vi "format_streaming_channels.set.vi"(8 "error in":errorcluster, 9 "paths":string[](array[string]), 10 "names":string[](array[string]), 11 "Nominal IO Client in":T1 format="%.0x") -> (0 "error out":errorcluster, 1 "saved paths":string[](array[string]), 2 "saved names":string[](array[string]), 3 "Nominal IO Client out":T1 format="%.0x")   [LabVIEW 2024, in "Nominal Client Scripting.lvlib"]
uses:
  Nominal Client Scripting.lvlib
  <vilib>/NI VeriStand/Custom Device API/Custom Device Item Ref.ctl
  <vilib>/NI VeriStand/Custom Device API/Custom Device API.lvlib
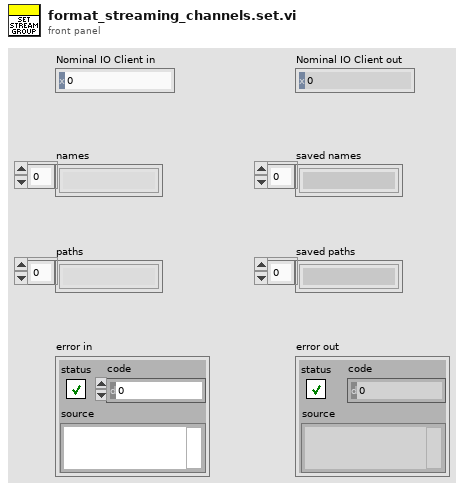
[diagram p1: front panel]
types:
  T1 = typedef "Custom Device API.lvlib/Custom Device Item Ref.ctl" = u64
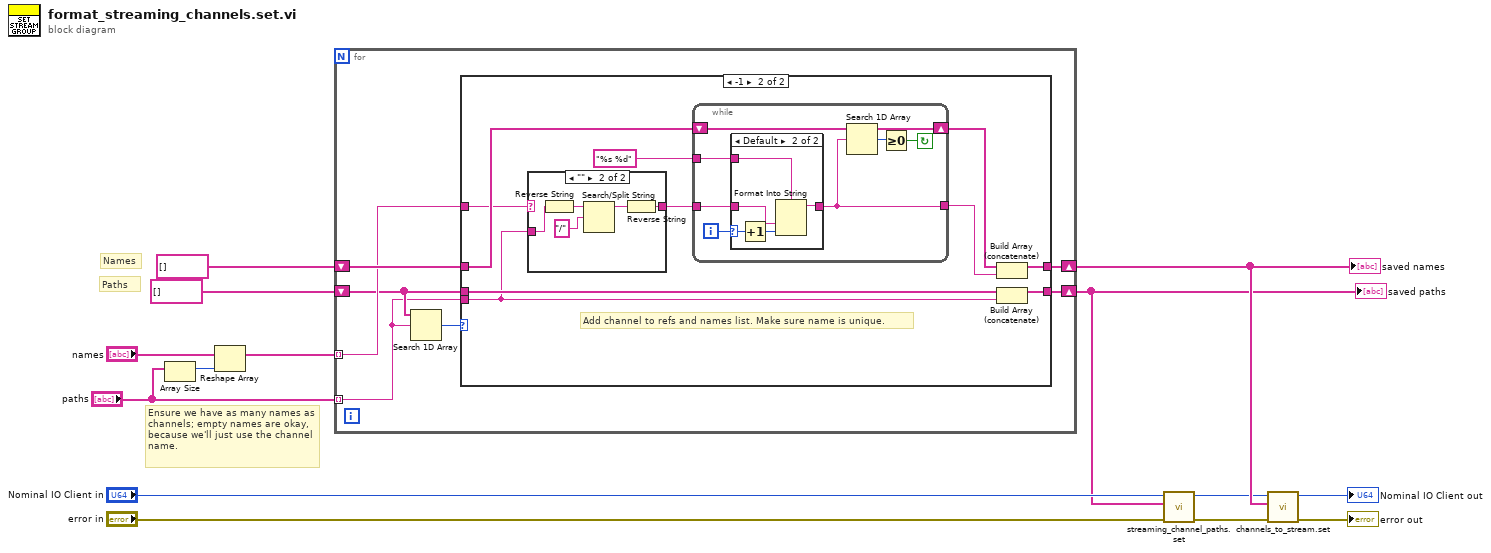
[diagram p0: block diagram]
diagram:
  # "Paths"
  # "Names"
  # "Ensure we have as many names as channels; empty names are okay, because we'll just use the channel name."
  n1 = Array Size(array="paths") -> (size(s)=w11:i32)
  n2 = Reshape Array("names", w11) -> (w12:string[])
  n3 = for {
    shift-right: [w21] -> w4
    shift-left: string[] [] -> [w17]
    shift-right: [w19] -> w10
    shift-left: string[] [] -> [w20]
    tunnel: "paths" -> [w15] mode=indexing
    tunnel: w12 -> [w18] mode=indexing
    n4 = Search 1D Array(1D array=w17, element=w15) -> (index of element=w16:i32)  [unwired: 1 out]
    n5 = case shown="-1" w16 {
      tunnel: w17 -> [w23 w33]
      tunnel: [w23 w32] -> w21
      tunnel: w15 -> [_ w31]
      tunnel: w20 -> [w22 w27]
      tunnel: [w22 w30] -> w19
      tunnel: w18 -> [_ w24]
      frame Default {
        # "Channel already selected for logging. Don't add to refs or names list."
      }
      frame -1 {
        # "Add channel to refs and names list. Make sure name is unique."
        n6 = case shown="\"\"" w24 {
          selector: w24 -> [w34 _]
          tunnel: w31 -> [_ w39]
          tunnel: [w34 w35] -> w26
          frame Default {
          }
          frame "" {
            n7 = Reverse String(1:w39) -> (0:w38:string)
            n8 = Search/Split String(string=w38, search string/char (-)="/") -> (substring before match=w36:string)  [unwired: 1 in, 2 out]
            n9 = Reverse String(1:w36) -> (0:w35:string)
          }
        }
        n10 = while {
          shift-right: [w44] -> w28
          shift-left: w27 -> [w44]
          tunnel: w26 -> [w45]
          tunnel: [w41] -> w25
          tunnel: "%s %d" ("format string") -> [w40]
          i -> [w46]
          stop <- w42 continue-if-true
          n11 = case shown="Default" w46 {
            selector: w46 -> [_ w50]
            tunnel: w45 -> [w47 w48]
            tunnel: [w47 w52] -> w41
            tunnel: w40 -> [_ w51]
            frame 0 {
            }
            frame Default {
              n12 = Increment(x=w50) -> (x+1=w49:i32)
              n13 = Format Into String(format string=w51, w48, w49) -> (resulting string=w52:string)  [unwired: 2 in, 1 out]
            }
          }
          n14 = Search 1D Array(1D array=w44, element=w41) -> (index of element=w43:i32)  [unwired: 1 out]
          n15 = Greater Or Equal To 0?(x=w43) -> (x >= 0?=w42:bool)
        }
        n16 = Build Array (concatenate)(w28, w25) -> (w30:string[])
        n17 = Build Array (concatenate)(w33, w31) -> (w32:string[])
      }
    }
  }
  "saved names" <- w10
  "saved paths" <- w4
  n18 = call "streaming_channel_paths.set.vi"("error in (no error)"="error in", "Channel Paths"=w4, "Item Ref in"="Nominal IO Client in") -> ("error out"=w2:errorcluster, "Item Ref out"=w1:T1)  [unwired: 7 in]
  n19 = call "channels_to_stream.set.vi"("error in (no error)"=w2, "Channels to Stream"=w10, "Nominal IO Client in"=w1) -> ("error out"=→"error out":errorcluster, "Nominal IO Client out"=→"Nominal IO Client out":T1)  [unwired: 6 in, 1 out]
